vi "BangBang_SetTolerance.vi"(10 "Tolerance":dbl, 11 "BANG_BANG":T1 {"Measurment" format="%13.5p"; "Setpoint" format="%13.5p"; "Tolerance" format="%13.5p"}) -> (3 "out BANG_BANG":T1 {"Measurment" format="%13.5p"; "Setpoint" format="%13.5p"; "Tolerance" format="%13.5p"})   [LabVIEW 2019, in "Trajectory_Library.lvlib"]
doc: "Sets the error within which atSetpoint will return true.\n \n \nInput:\n - BangBang -- Data cluster\n - tolerance -- Position error which is tolerable.\n\nOutput\n - outBangBang -- Updated data cluster"
uses:
  Trajectory_Library.lvlib
  TypeDef/BANG_BANG.ctl
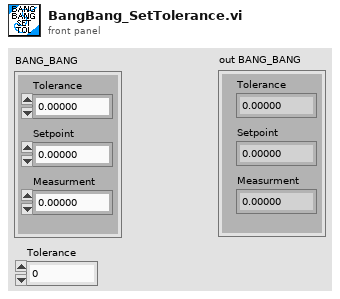
[diagram p1: front panel]
types:
  T1 = typedef "Trajectory_Library.lvlib/BANG_BANG.ctl" = cluster{"Tolerance":dbl, "Setpoint":dbl, "Measurment":dbl}
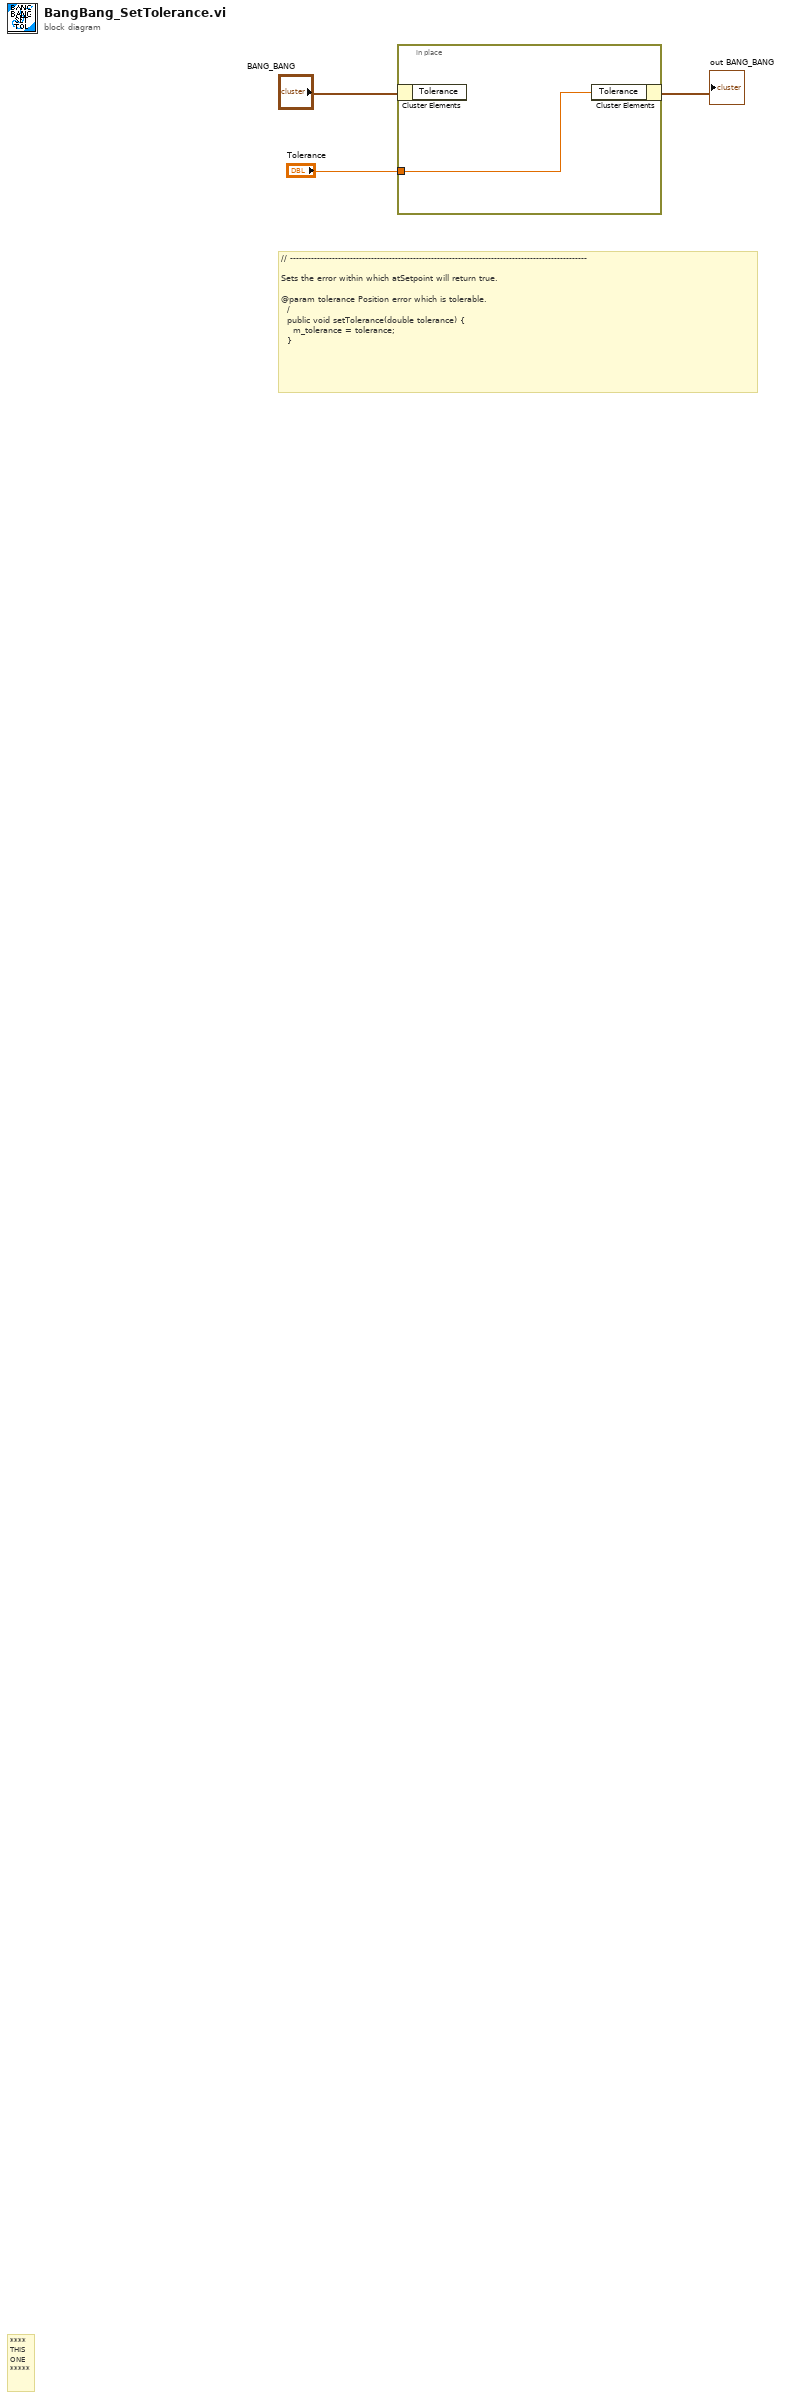
[diagram p0: block diagram]
diagram:
  # "// ---------------------------------------------------------------------------------------------------\n  \nSets the error within which atSetpoint will return true.\n  \n@param tolerance Position error which is tolerable.\n  /\n  public void setTolerance(double tolerance) {\n    m_tolerance = tolerance;\n  }"
  # "****\nTHIS\nONE\n*****"
  n1 = in-place {
    in-place-border: "Tolerance" -> [w4]
    n2 = in-place-cluster #1("BANG_BANG") -> ()  [unwired: 1 out]
    n3 = in-place-cluster #1("Tolerance"=w4) -> (→"out BANG_BANG":T1)
  }
